vi "Status LED.vi"(9 "Fehler":bool, 10 "Aktiv":bool, 11 "Boolean (Eingang)":refnum<vi>) -> ()   [LabVIEW 2020, in "Backup.lvlib"]
uses:
  Backup.lvlib
panel:
  out "Farben [4]":cluster{u32, u32}[](array[cluster])
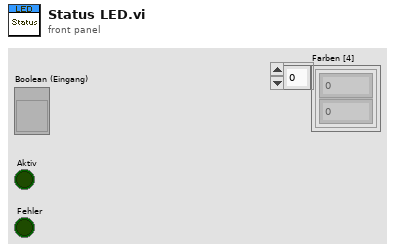
[diagram p1: front panel]
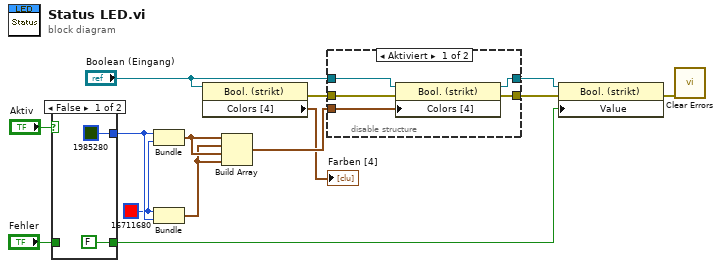
[diagram p0: block diagram]
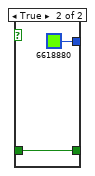
[diagram p3: hidden frame]
diagram:
  w5 = u32 16711680
  n1 = case shown="False" "Aktiv" {
    tunnel: [u32 1985280 u32 6618880] -> w6
    tunnel: [FALSE w17] -> w2
    tunnel: "Fehler" -> [_ w17]
    frame False {
    }
    frame True {
    }
  }
  n2 = Bundle(w6, w5) -> (w4:cluster{u32, u32})  [unwired: 1 in]
  n3 = Bundle(w5, w6) -> (w3:cluster{u32, u32})  [unwired: 1 in]
  n4 = property class="Bool. (strikt)"(reference="Boolean (Eingang)") -> (error out=w7:errorcluster, "Colors [4]"=→"Farben [4]":cluster{u32, u32}[])  [unwired: 1 in, 1 out]
  n5 = Build Array(w4, w3, w4, w3) -> (w13:cluster{u32, u32}[])
  n6 = disable-structure shown="Aktiviert" {
    disable-tunnel: w13 -> [w23 _]
    disable-tunnel: [w22 w25] -> w12
    disable-tunnel: [w21 w24] -> w11
    disable-tunnel: "Boolean (Eingang)" -> [w20 w25]
    disable-tunnel: w7 -> [w19 w24]
    frame Enabled {
      n7 = property class="Bool. (strikt)"(reference=w20, error in=w19, "Colors [4]"=w23) -> (reference out=w22:refnum<vi>, error out=w21:errorcluster)
    }
    frame Disabled {
    }
  }
  n8 = property class="Bool. (strikt)"(reference=w12, error in=w11, "Value"=w2) -> (error out=w10:errorcluster)  [unwired: 1 out]
  n9 = call <vilib>:"Clear Errors.vi"("error in (no error)"=w10) -> ()  [unwired: 5 in, 2 out]
